vi "Set Max Meter ROI.vi"(8 "error in (no error)":errorcluster, 10 "ROI":T2, 11 "Item Ref in":T1 format="%.0x") -> (0 "error out":errorcluster, 3 "Item Ref out":T1 format="%.0x")   [LabVIEW 2011, in "Meter Detection Custom Device.lvlib"]
uses:
  Meter Detection Custom Device.lvlib
  <vilib>/NI Veristand/Custom Device API/Custom Device Item Ref.ctl
  Meter Detection Global Variable.vi
  <vilib>/NI Veristand/Custom Device API/Set Item Property (Variant).vi
  <vilib>/NI Veristand/Custom Device API/Custom Device API.lvlib
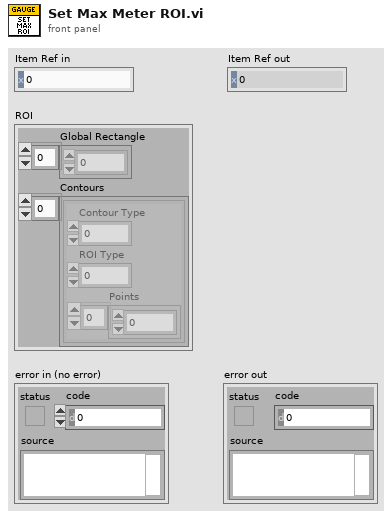
[diagram p1: front panel]
types:
  T1 = typedef "Custom Device API.lvlib/Custom Device Item Ref.ctl" = u64
  T2 = cluster{"Global Rectangle":i32[], "Contours":cluster{"Contour Type":u32, "ROI Type":u32, "Points":i32[]}[]}
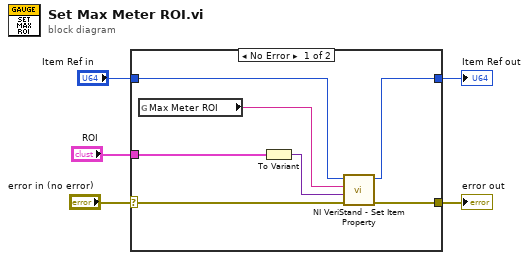
[diagram p0: block diagram]
diagram:
  n1 = case shown="No Error" "error in (no error)" {
    selector: "error in (no error)" -> [w6 w14]
    tunnel: [w11 w14] -> w5
    tunnel: "Item Ref in" -> [w10 w13]
    tunnel: "ROI" -> [w8 _]
    tunnel: [w7 w13] -> w2
    frame No Error {
      n2 = global read "Meter Detection Global Variable.vi" "Max Meter ROI"() -> (w9:string)
      n3 = To Variant(anything=w8) -> (Variant=w12:variant)
      n4 = call-poly <vilib>:"NI VeriStand - Set Item Property.vi"("error in (no error)"=w6, "Value"=w12, "Property Name"=w9, "Item Ref in"=w10) -> ("error out"=w11:errorcluster, "Item Ref out"=w7:T1)  [unwired: 5 in, 1 out]
    }
    frame Error {
    }
  }
  "error out" <- w5
  "Item Ref out" <- w2
